vi "FPGA Counts.vi"(0 "saveData":bool, 2 "runs":i32, 5 "fpgaCommand":u8, 7 "fileName":string, 11 "error in (no error)":errorcluster) -> (4 "function return":i32, 12 "data":i64[](array[numeric]), 13 "stats":i64[](array[numeric]), 14 "length":i32, 15 "error out":errorcluster)   [LabVIEW 2012, in "Stats.lvlib"]
doc: "Count clicks and coincidences on four channels with a Xylo-EM FPGA board.\n\nLIBRARY_API int FPGA_Counts(bool saveData, unsigned char fpgaCommand,char* fileName, int* data, int* length, int runs);\n\nLIBRARY_API int FPGA_Counts(bool saveData, unsigned char fpgaCommand, char* fileName, int* stats, unsigned int* data, int* length, int runs);\n\nLIBRARY_API int FPGA_Counts(bool saveData, unsigned char fpgaCommand, char* fileName, __int64* stats, unsigned __int64* data, int* length, int runs);"
uses:
  Stats.lvlib
  Stats/Release/x64/Stats.dll
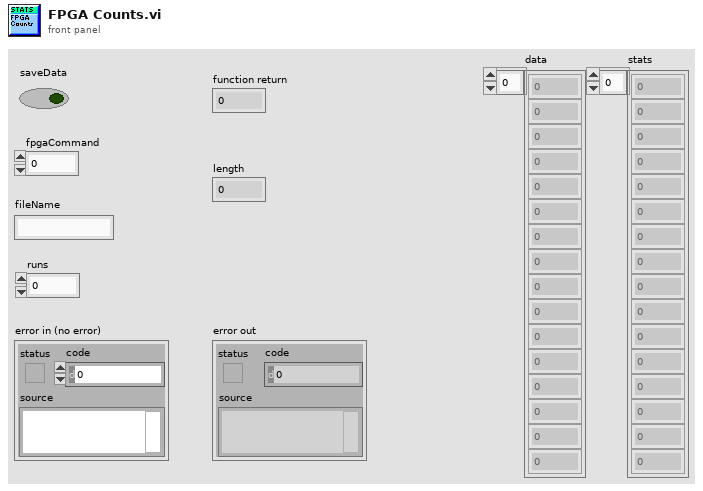
[diagram p1: front panel]
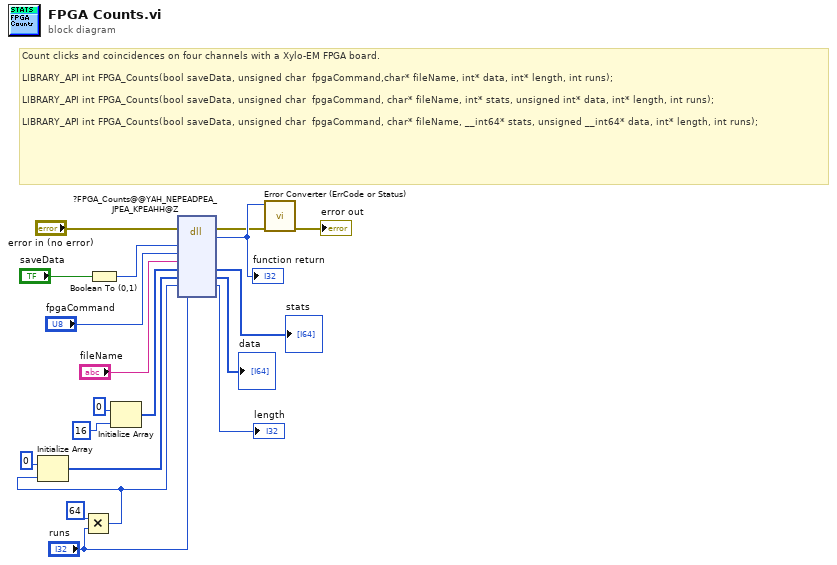
[diagram p0: block diagram]
diagram:
  # "Count clicks and coincidences on four channels with a Xylo-EM FPGA board.\n\nLIBRARY_API int FPGA_Counts(bool saveData, unsigned char  fpgaCommand,char* fileName, int* data, int* length, int runs);\n\nLIBRARY_API int FPGA_Counts(bool saveData, unsigned char  fpgaCommand, char* fileName, int* stats, unsigned int* data, int* length, int runs);\n\nLIBRARY_API int FPGA_Counts(bool saveData, unsigned char  fpgaCommand, char* fileName, __int64* stats, unsigned __int64* data, int* length, int runs);"
  n1 = Multiply(x=64, y="runs") -> (x*y=w2:i32)
  n2 = Initialize Array(0, w2) -> (w5:i32[])
  n3 = Boolean To (0,1)(Boolean="saveData") -> (0, 1=w17:i16)
  n4 = Initialize Array(0, 16) -> (w7:i32[])
  n5 = dll-call lib="C:/Programming/Stats/Stats/Release/x64/Stats.*" fn="?FPGA_Counts@@YAH_NEPEADPEA_JPEA_KPEAHH@Z"(error in="error in (no error)", "saveData"=w17, "fpgaCommand"="fpgaCommand", "fileName"="fileName", "stats"=w7, "data"=w5, "length"=w2, "runs"="runs") -> (error out=w13:errorcluster, "return type"=w19:i32, "stats"=→"stats":i64[], "data"=→"data":u64[], "length"=→"length":i32)  [unwired: 6 in, 1 out]
  "function return" <- w19
  n6 = call "Error Converter (ErrCode or Status).vi"("error in (no error)"=w13, "error code"=w19) -> ("error out"=→"error out":errorcluster)  [unwired: 9 in]
